vi "计算标准坐标在影像坐标系坐标.vi"(0 "Angle":dbl, 1 "参考点影像坐标":cluster{"X":sgl, "Y":sgl}, 2 "标准点坐标输入":cluster{"Distance":dbl, "Distance":dbl}[](array[cluster]), 3 "第一个点与参考点在产品坐标系位置差":cluster{"X":sgl, "Y":sgl}={"X"=-237.0, "Y"=135.0}) -> (7 "标准的影像坐标":cluster{dbl, dbl}[](array[cluster]))   [LabVIEW 2014]
uses:
  <vilib>/Analysis/coordinate.llb/2D Cartesian Coordinate Rotation (Scalar).vi
  <vilib>/Analysis/NI_AALPro.lvlib
panel:
  out "第一个点的影像坐标":cluster{dbl, dbl}
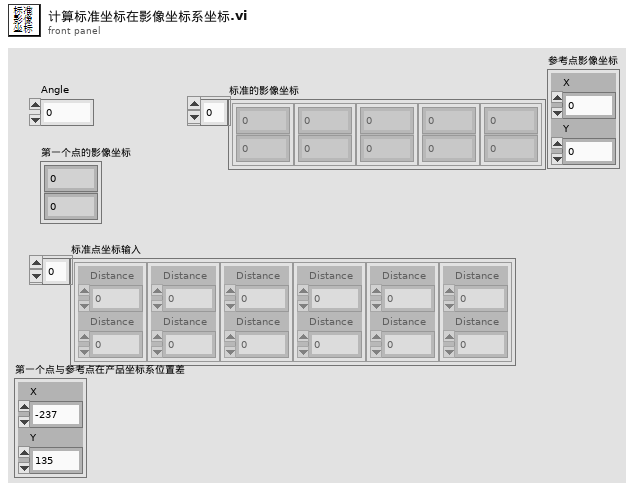
[diagram p1: front panel]
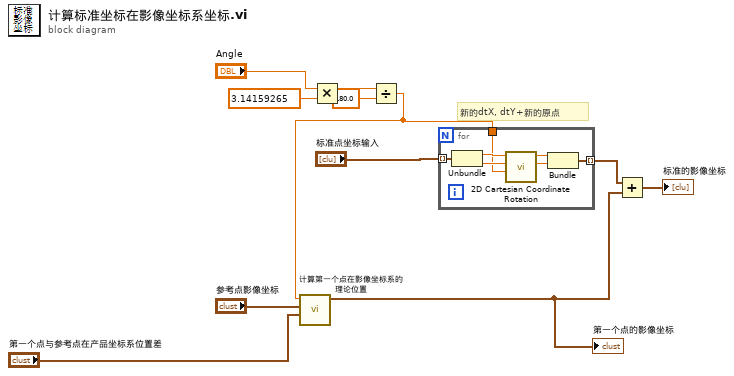
[diagram p0: block diagram]
diagram:
  # "新的dtX, dtY+新的原点"
  n1 = Multiply(x="Angle", y=3.14159265) -> (x*y=w6:dbl)
  n2 = Divide(x=w6, y=180.0) -> (x/y=w3:dbl)
  n3 = call "计算第一个点在影像坐标系的理论位置.vi"("第一个点与参考点在产品坐标系位置差"="第一个点与参考点在产品坐标系位置差", "参考点影像坐标"="参考点影像坐标", "Angle (Pixel)"=w3) -> ("第一个点在影像坐标系坐标"=w1:cluster{dbl, dbl})  [unwired: 8 in]
  "第一个点的影像坐标" <- w1
  n4 = for {
    tunnel: w3 -> [w12]
    tunnel: "标准点坐标输入" -> [w18] mode=indexing
    tunnel: [w13] -> w10 mode=indexing
    n5 = Unbundle(w18) -> ("Distance"=w17:dbl, "Distance"=w16:dbl)
    n6 = call-poly <vilib>:"2D Cartesian Coordinate Rotation.vi"("theta"=w12, "y"=w16, "x"=w17) -> ("y out"=w14:dbl, "x out"=w15:dbl)  [unwired: 6 in, 1 out]
    n7 = Bundle("x out"=w15, "y out"=w14) -> (w13:cluster{"x out":dbl, "y out":dbl})  [unwired: 1 in]
  }
  n8 = Add(x=w10, y=w1) -> (x+y=→"标准的影像坐标":cluster{dbl, dbl}[])
